vi "Teleop Intake Control.vi"() -> ()   [LabVIEW 2016]
uses:
  Common Code/Gamepads/Axes Cluster.ctl
  Common Code/Gamepads/Button Cluster.ctl
  Common Code/Gamepads/D-Pad.ctl
  Common Code/Intake Commands.ctl
  Common Code/Utilities/Change Detect Boolean.vi
  Robot Global Data.vi
panel:
  in  "D-Pad":T1
  in  "Button Cluster":T2
  in  "Axes":T3
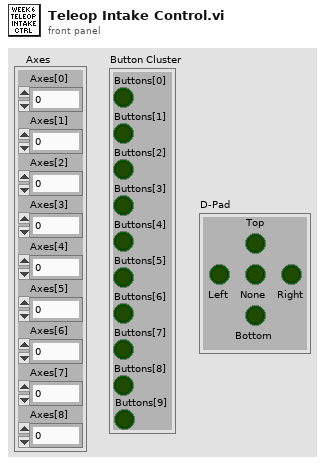
[diagram p1: front panel]
types:
  T1 = typedef "D-Pad.ctl" = cluster{"Top":bool, "Bottom":bool, "None":bool, "Right":bool, "Left":bool}
  T2 = typedef "Button Cluster.ctl" = cluster{"Buttons[0]":bool, "Buttons[1]":bool, "Buttons[2]":bool, "Buttons[3]":bool, "Buttons[4]":bool, "Buttons[5]":bool, "Buttons[6]":bool, "Buttons[7]":bool, "Buttons[8]":bool, "Buttons[9]":bool}
  T3 = typedef "Axes Cluster.ctl" = cluster{"Axes[0]":dbl, "Axes[1]":dbl, "Axes[2]":dbl, "Axes[3]":dbl, "Axes[4]":dbl, "Axes[5]":dbl, "Axes[6]":dbl, "Axes[7]":dbl, "Axes[8]":dbl}
  T4 = typedef "Intake Mode.ctl" = enum16{"Manual", "Auto"}
  T5 = typedef "Intake Commands.ctl" = enum16{"Idle", "Intake", "Outtake"}
  T6 = typedef "Intake Command Cluster.ctl" = cluster{"Intake Mode":T4, "Intake Command":T5, "Intake Manual Power":dbl}
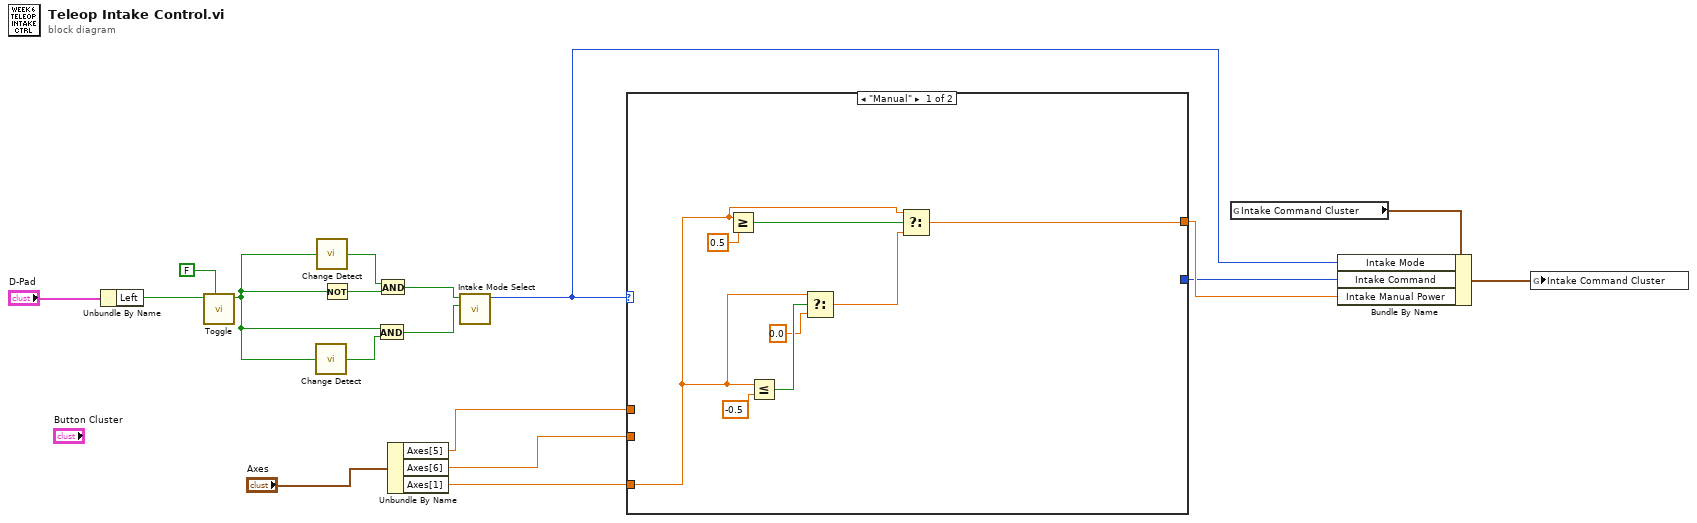
[diagram p0: block diagram]
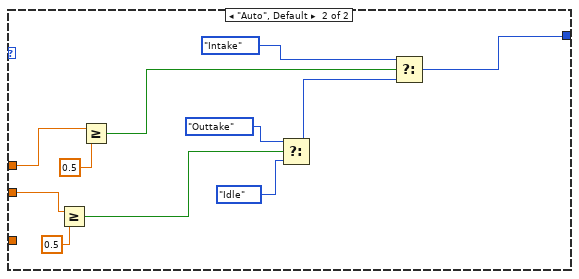
[diagram p2: hidden frame]
diagram:
  n1 = Unbundle By Name("D-Pad") -> ("Left"=w16:bool)
  n2 = call "Toggle.vi"("Initial Value"=FALSE, "In"=w16) -> ("Toggled"=w11:bool)  [unwired: 9 in]
  n3 = call-poly "Change Detect.vi"("In"=w11) -> ("Changed?"=w12:bool)
  n4 = call-poly "Change Detect.vi"("In"=w11) -> ("Changed?"=w13:bool)
  n5 = Not(x=w11) -> (.not. x?=w14:bool)
  n6 = And(x=w11, y=w12) -> (x .and. y?=w9:bool)
  n7 = And(x=w13, y=w14) -> (x .and. y?=w10:bool)
  n8 = Unbundle By Name("Axes") -> ("Axes[5]"=w6:dbl, "Axes[6]"=w5:dbl, "Axes[1]"=w8:dbl)
  n9 = call "Intake Mode Select.vi"("Manual"=w9, "Auto"=w10) -> ("Intake Mode"=w3:T4)  [unwired: 9 in]
  n10 = case shown="\"Manual\"" w3 {
    tunnel: w8 -> [w20 _]
    tunnel: [w19 _] -> w7
    tunnel: w6 -> [_ w35]
    tunnel: w5 -> [_ w34]
    tunnel: [_ w27] -> w4
    frame "Manual" {
      n11 = Greater Or Equal?(x=w20, y=0.5) -> (x >= y?=w24:bool)
      n12 = Less Or Equal?(x=w20, y=-0.5) -> (x <= y?=w22:bool)
      n13 = Select(t=w20, s=w22, f=0.0) -> (s? t:f=w23:dbl)
      n14 = Select(t=w20, s=w24, f=w23) -> (s? t:f=w19:dbl)
    }
    frame "Auto", Default {
      n15 = Greater Or Equal?(x=w34, y=0.5) -> (x >= y?=w32:bool)
      n16 = Greater Or Equal?(x=w35, y=0.5) -> (x >= y?=w33:bool)
      n17 = Select(t=Intake_Commands."Outtake" ("Intake Command"), s=w32, f=Intake_Commands."Idle" ("Intake Command")) -> (s? t:f=w29:T5)
      n18 = Select(t=Intake_Commands."Intake" ("Intake Command"), s=w33, f=w29) -> (s? t:f=w27:T5)
    }
  }
  n19 = global read "Robot Global Data.vi" "Intake Command Cluster"() -> (w17:T6)
  n20 = Bundle By Name(cluster=w17, "Intake Mode"=w3, "Intake Command"=w4, "Intake Manual Power"=w7) -> (w18:T6)
  n21 = global write "Robot Global Data.vi" "Intake Command Cluster"(w18) -> ()
